vi "CPP-ScanTimeKeeper.vi"(4 "Scan Period":dbl format="%.2f", 5 "Previous Scan Value":dbl format="%.2f", 6 "Present scan array":dbl[](array[numeric]) format="%.2f", 7 "Value to Output":dbl format="%.2f", 8 "Ch Description":T1={"Ch Name"="ADAM:Scan:Time", "Type"="Hold Value", "Function"=enum."Analogue Input", "Ch State"=enum."On", "Calibration type"=enum."Raw", "A"=0.0, "B"=0.0, "C"=0.0, "D"=0.0, "Comments"="", "Address"={"Main"=0, "Ch."=0, "Sub"=0, "Port Name"=""}, "String"="", "Duty"=65535} {"Duty" format="%.0b"; "D" format="%#_5g"; "C" format="%#_5g"; "B" format="%#_5g"; "A" format="%#_5g"}, 9 "Ch names":string[](array[string])) -> (0 "Scan comment":string, 1 "Output":dbl=3523369712.9230537 format="%.3f")   [LabVIEW 2014]
uses:
  ADAM Client/Sub VIs/ADAM Controls/Ch_description_ADAM.ctl
  ADAM Client/Sub VIs/ADAM Controls/Module_type_ADAM.ctl
  ADAM Client/Sub VIs/ADAM Controls/Function_ADAM.ctl
  ADAM Client/Sub VIs/ADAM Controls/Channel_State.ctl
  ADAM Client/Sub VIs/ADAM Controls/Calib_type_ADAM.ctl
  ADAM Client/Sub VIs/ADAM Controls/Address.ctl
panel:
  out "D":dbl format="%#.1f"
  out "C 2":dbl format="%#.1f"
  out "C":dbl format="%#.1f"
  out "current time":timestamp
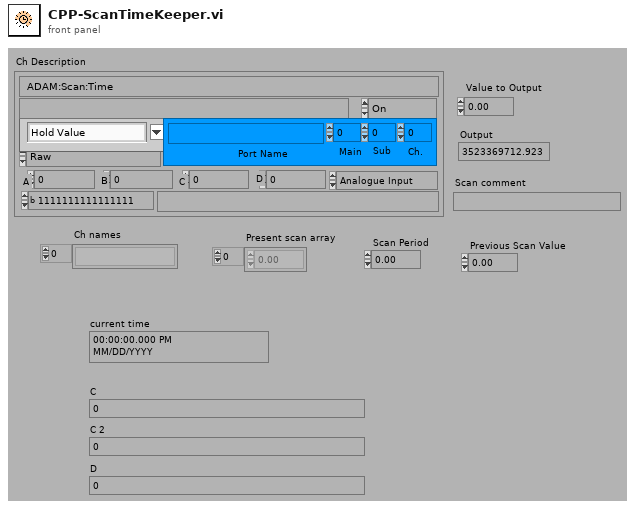
[diagram p1: front panel]
types:
  T1 = typedef "Ch_description_ADAM.ctl" = cluster{"Ch Name":string, "Type":T2, "Function":T3, "Ch State":T4, "Calibration type":T5, "A":dbl, "B":dbl, "C":dbl, "D":dbl, "Comments":string, "Address":T6, "String":string, "Duty":u16}
  T2 = typedef "Module_type_ADAM.ctl" = string
  T3 = typedef "Function_ADAM.ctl" = enum16{"Analogue Input", "Digital Input", "Event counter", "Event rate", "Analogue Output", "Digital Output", "Relay Output"}
  T4 = typedef "Channel_State.ctl" = enum16{"On", "Off", "Always On", "Always Off"}
  T5 = typedef "Calib_type_ADAM.ctl" = enum16{"Raw", "Bx + A", "Cx^2 + Bx + A", "Dx^3 + Cx^2 + Bx + A", "In Band", "Hi-Tec Q", "Hi-Tec M_dot", "Text"}
  T6 = typedef "Address.ctl" = cluster{"Main":i32, "Ch.":i32, "Sub":i32, "Port Name":string}
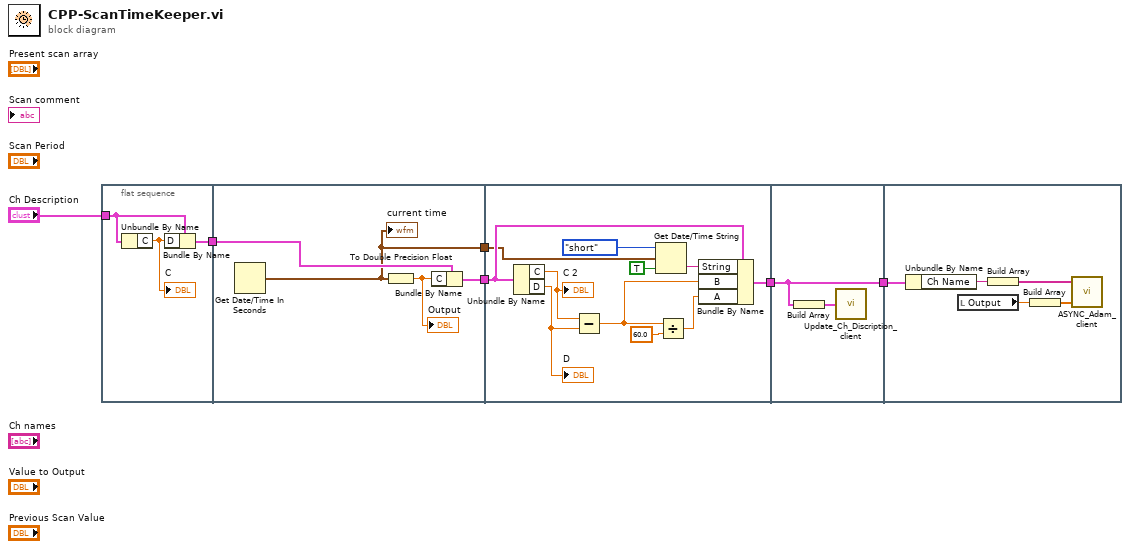
[diagram p0: block diagram]
diagram:
  n1 = flat-sequence {
    tunnel: "Ch Description" -> [w8]
    tunnel: [w7] -> w5
    tunnel: w5 -> [w13]
    tunnel: [w12] -> w4
    tunnel: [w11] -> w3
    tunnel: w4 -> [w18]
    tunnel: w3 -> [w16]
    tunnel: [w15] -> w2
    tunnel: w2 -> [w25]
    tunnel: [w25] -> w1
    tunnel: w1 -> [w29]
    frame #0 {
      n2 = Unbundle By Name(w8) -> ("C"=w9:dbl)
      "C" <- w9
      n3 = Bundle By Name(cluster=w8, "D"=w9) -> (w7:T1)
    }
    frame #1 {
      n4 = Get Date/Time In Seconds() -> (seconds since 1Jan1904=w11:timestamp)
      "current time" <- w11
      n5 = To Double Precision Float(number=w11) -> (double precision float=w10:dbl)
      "Output" <- w10
      n6 = Bundle By Name(cluster=w13, "C"=w10) -> (w12:T1)
    }
    frame #2 {
      n7 = Unbundle By Name(w18) -> ("C"=w24:dbl, "D"=w23:dbl)
      "C 2" <- w24
      "D" <- w23
      n8 = Subtract(x=w24, y=w23) -> (x-y=w14:dbl)
      n9 = Get Date/Time String(date format (0)=enum16{"short", "long", "abbreviated"}."short", seconds (now)=w16, want seconds? (F)=TRUE) -> (time string=w17:string)  [unwired: 1 out]
      n10 = Divide(x=w14, y=60.0) -> (x/y=w21:dbl)
      n11 = Bundle By Name(cluster=w18, "String"=w17, "B"=w14, "A"=w21) -> (w15:T1)
    }
    frame #3 {
      n12 = Build Array(w25) -> (w26:T1[])
      n13 = call "Update_Ch_Discription_client.vi"("Channels to update In"=w26) -> ()  [unwired: 1 out]
    }
    frame #4 {
      n14 = Unbundle By Name(w29) -> ("Ch Name"=w28:string)
      n15 = local read "Output"() -> (w31:dbl)
      n16 = Build Array(w28) -> (w27:string[])
      n17 = Build Array(w31) -> (w30:dbl[])
      n18 = call "ASYNC_Adam_client.vi"("Values"=w30, "Channel Names"=w27) -> ()  [unwired: 1 in, 2 out]
    }
  }
